vi "StepApproach.vi"() -> ()   [LabVIEW 2014]
uses:
  <vilib>/rvi/eio/common/nirviEmuTemplateMethod_errors.vi
  <vilib>/rvi/Emulation/niFpgaGetClockAttributes.vi
  <vilib>/rvi/Emulation/niFpgaSctlEmulationGetInTimedLoop.vi
  <vilib>/rvi/Emulation/niFpgaEmulationReportErrorSimple.vi
  <vilib>/rvi/Emulation/niFpgaCriticalErrorInLSC.vi
  <vilib>/rvi/Emulation/niFpgaProcessEmulError.vi
  <vilib>/rvi/interface/RandomDataEmulation/niFpgaRandomDataHandleErrors.vi
  <vilib>/eio/EIONode/EIONode.xnode
  <vilib>/rvi/DataTransferAndStorage/Container/XNode/niFpgaContainer.xnode
  <vilib>/rvi/interface/RandomDataEmulation/nirviRandomDataFpgaReadWriteTemplate.vi
panel:
  out "Numeric":i16
  out "PresentCount":i32
  in  "MeasureCount":i16
  in  "SeveralSampleMeasure?":bool
  in  "WithdrawStep":i16
  out "Result":bool
  out "PIZPosIndexDia":i16(graph)
  out "PreCurrIndexDia":i16(graph)
  out "PIZMaxPosIndex":i16
  out "PIZPosIndex":i16
  in  "stop":bool
  out "Approached?":bool
  in  "Offset":i16
  in  "AppRate us":u32
  out "RealPosIndex":i16
  out "preCurrIndex":i16
  in  "Percentage %":sgl format="%#_13g"
  in  "CurrSampleNum":u32
  in  "BaseTime us":u32
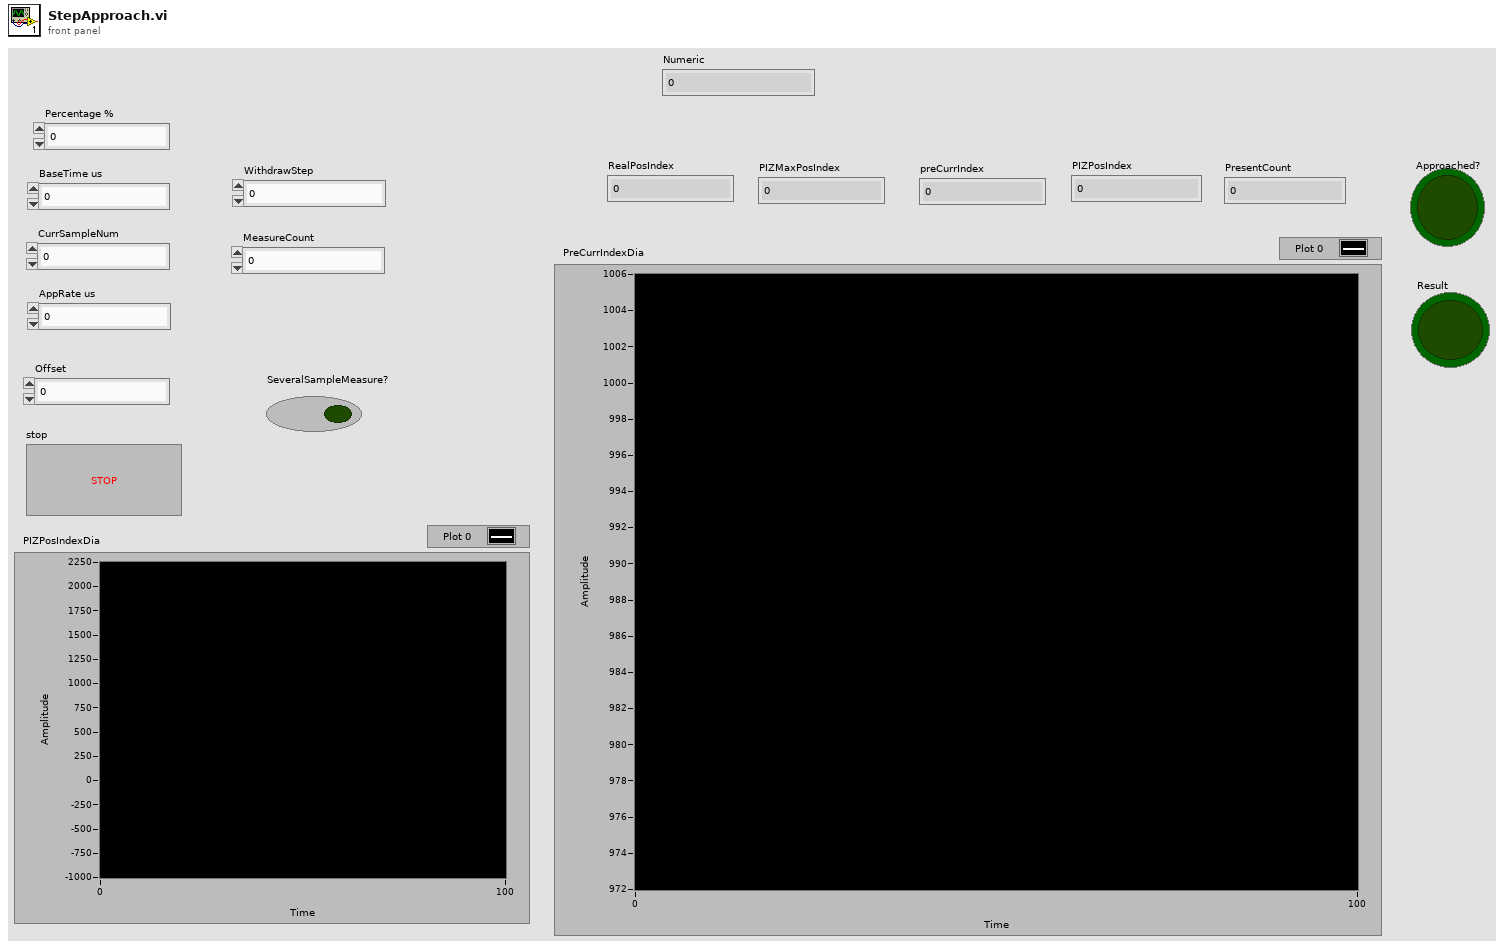
[diagram p1: front panel]
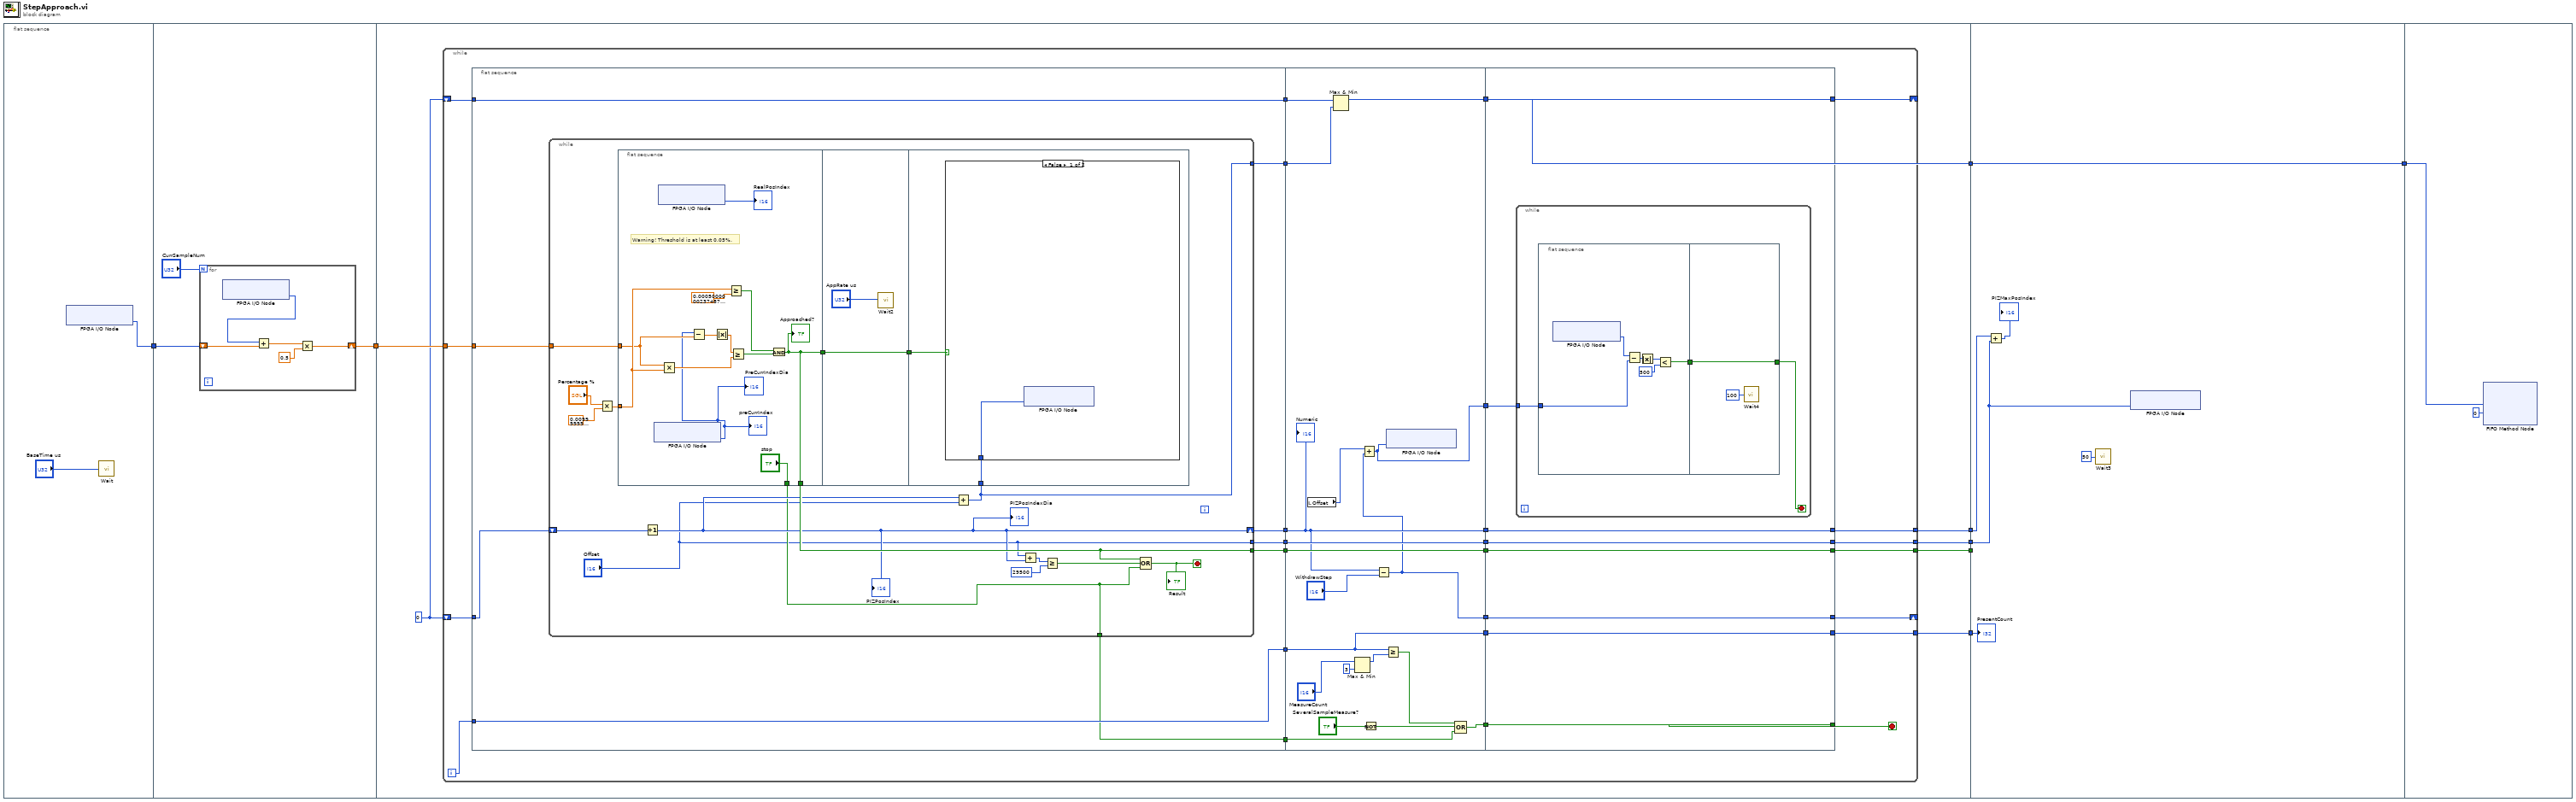
[diagram p0: block diagram]
diagram:
  n1 = flat-sequence {
    tunnel: [w9] -> w8
    tunnel: w8 -> [w12]
    tunnel: [w11] -> w7
    tunnel: w7 -> [w25]
    tunnel: [w24] -> w6
    tunnel: [w23] -> w5
    tunnel: [w22] -> w4
    tunnel: [w20] -> w3
    tunnel: [w21] -> w1
    tunnel: w6 -> [_]
    tunnel: w5 -> [w134]
    tunnel: w4 -> [w135]
    tunnel: w3 -> [w137]
    tunnel: [w137] -> w2
    tunnel: w1 -> [w132]
    tunnel: w2 -> [w139]
    frame #0 {
      n2 = xnode "FPGA I/O Node"() -> ("Connector0/AI1"=w9:i16)  [unwired: 1 in, 1 out]
      n3 = call "Wait"("Count(uSec)"="BaseTime us") -> ()  [unwired: 1 out]
    }
    frame #1 {
      n4 = for {
        N: "CurrSampleNum" -> [_]
        shift-right: [w14] -> w11
        shift-left: w12 -> [w17]
        n5 = xnode "FPGA I/O Node"() -> ("Connector0/AI1"=w18:i16)  [unwired: 1 in, 1 out]
        n6 = Add(x=w18, y=w17) -> (x+y=w16:sgl)
        n7 = Multiply(x=w16, y=sgl 0.5) -> (x*y=w14:sgl)
      }
    }
    frame #2 {
      w19 = i16 0
      n8 = while {
        tunnel: w25 -> [w51]
        tunnel: [w50] -> w24
        tunnel: [w49] -> w23
        tunnel: [w48] -> w22
        shift-right: [w43] -> _
        shift-left: w19 -> [w42]
        tunnel: [w38] -> w21
        shift-right: [w36] -> w20
        shift-left: w19 -> [w35]
        i -> [w41]
        stop <- w39 stop-if-true
        n9 = flat-sequence {
          tunnel: w51 -> [w60]
          tunnel: w42 -> [w52]
          tunnel: [w59] -> w47
          tunnel: [w58] -> w46
          tunnel: [w57] -> w45
          tunnel: [w56] -> w44
          tunnel: w41 -> [w55]
          tunnel: [w55] -> w40
          tunnel: w35 -> [w54]
          tunnel: [w54] -> w37
          tunnel: [w53] -> w27
          tunnel: w47 -> [w112]
          tunnel: w46 -> [w111]
          tunnel: w45 -> [w110]
          tunnel: w44 -> [w102]
          tunnel: w40 -> [w104]
          tunnel: w37 -> [w103]
          tunnel: [w112] -> w34
          tunnel: [w111] -> w33
          tunnel: [w110] -> w32
          tunnel: [w95] -> w31
          tunnel: [w98] -> w30
          tunnel: [w104] -> w29
          tunnel: [w101] -> w28
          tunnel: w27 -> [w97]
          tunnel: [w94] -> w26
          tunnel: [w115] -> w36
          tunnel: [w116] -> w38
          tunnel: [w117] -> w39
          tunnel: [w114] -> w43
          tunnel: [w118] -> w48
          tunnel: [w119] -> w49
          tunnel: [w120] -> w50
          tunnel: w34 -> [w120]
          tunnel: w33 -> [w119]
          tunnel: w32 -> [w118]
          tunnel: w31 -> [w114]
          tunnel: w30 -> [w117]
          tunnel: w29 -> [w116]
          tunnel: w28 -> [w115]
          tunnel: w26 -> [w113]
          frame #0 {
            n10 = while {
              tunnel: w60 -> [w76]
              shift-right: [w68] -> w57
              shift-left: w52 -> [w73]
              tunnel: [w72] -> w59
              tunnel: ["Offset"] -> w58
              tunnel: [w64] -> w56
              tunnel: [w62] -> w53
              stop <- w63 stop-if-true
              n11 = Multiply(x="Percentage %", y=sgl 0.01) -> (x*y=w65:sgl)
              n12 = flat-sequence {
                tunnel: w76 -> [w78]
                tunnel: [w83] -> w75
                tunnel: [w83] -> w72
                tunnel: ["stop"] -> w62
                tunnel: w65 -> [w81]
                tunnel: w75 -> [w90]
                tunnel: [w90] -> w74
                tunnel: w74 -> [w92]
                tunnel: w64 -> [w91]
                frame #0 {
                  # "Warning! Threshold is at least 0.05%."
                  n13 = xnode "FPGA I/O Node"() -> ("Connector0/AI1"=w77:i16)  [unwired: 1 in, 1 out]
                  "preCurrIndex" <- w77
                  "PreCurrIndexDia" <- w77
                  n14 = xnode "FPGA I/O Node"() -> ("Connector0/AI0"=→"RealPosIndex":i16)  [unwired: 1 in, 1 out]
                  n15 = Multiply(x=w78, y=w81) -> (x*y=w86:sgl)
                  n16 = Subtract(x=w77, y=w78) -> (x-y=w88:sgl)
                  n17 = Absolute Value(x=w88) -> (abs(x)=w87:sgl)
                  n18 = Greater Or Equal?(x=w81, y=sgl 0.0005) -> (x >= y?=w79:bool)
                  n19 = Greater Or Equal?(x=w87, y=w86) -> (x >= y?=w82:bool)
                  n20 = And(x=w79, y=w82) -> (x .and. y?=w83:bool)
                  "Approached?" <- w83
                }
                frame #1 {
                  n21 = call "Wait2"("Count(uSec)"="AppRate us") -> ()  [unwired: 1 out]
                }
                frame #2 {
                  n22 = case shown="False" w92 {
                    tunnel: w91 -> [w93 _]
                    frame False {
                      n23 = xnode "FPGA I/O Node"("Connector0/AO0"=w93) -> ()  [unwired: 1 in, 1 out]
                    }
                    frame True {
                    }
                  }
                }
              }
              n24 = Increment(x=w73) -> (x+1=w68:i16)
              "PIZPosIndex" <- w68
              "PIZPosIndexDia" <- w68
              n25 = Add(x=w68, y="Offset") -> (x+y=w64:i16)
              n26 = Add(x="Offset", y=w68) -> (x+y=w69:i16)
              n27 = Greater Or Equal?(x=w69, y=i16 29500) -> (x >= y?=w71:bool)
              n28 = Compound Arithmetic op=OR(w72, w71, w62) -> (w63:bool)
              "Result" <- w63
            }
          }
          frame #1 {
            n29 = local read "Offset"() -> (w96:i16)
            n30 = Max & Min(x=w103, y=w102) -> (max(x,y)=w101:i16)  [unwired: 1 out]
            n31 = Max & Min(x="MeasureCount", y=i16 3) -> (max(x,y)=w105:i16)  [unwired: 1 out]
            n32 = Not(x="SeveralSampleMeasure?") -> (.not. x?=w100:bool)
            n33 = Subtract(x=w110, y="WithdrawStep") -> (x-y=w95:i16)
            n34 = Add(x=w96, y=w95) -> (x+y=w94:i16)
            n35 = Greater Or Equal?(x=w104, y=w105) -> (x >= y?=w99:bool)
            n36 = xnode "FPGA I/O Node"("Connector0/AO0"=w94) -> ()  [unwired: 1 in, 1 out]
            n37 = Compound Arithmetic op=OR(w99, w100, w97) -> (w98:bool)
            "Numeric" <- w110
          }
          frame #2 {
            n38 = while {
              tunnel: w113 -> [w123]
              stop <- w122 stop-if-true
              n39 = flat-sequence {
                tunnel: w123 -> [w128]
                tunnel: [w126] -> w121
                tunnel: [w131] -> w122
                tunnel: w121 -> [w131]
                frame #0 {
                  n40 = xnode "FPGA I/O Node"() -> ("Connector0/AI0"=w129:i16)  [unwired: 1 in, 1 out]
                  n41 = Subtract(x=w129, y=w128) -> (x-y=w125:i16)
                  n42 = Absolute Value(x=w125) -> (abs(x)=w124:i16)
                  n43 = Less?(x=w124, y=i16 500) -> (x < y?=w126:bool)
                }
                frame #1 {
                  n44 = call "Wait4"("Count(uSec)"=u32 100) -> ()  [unwired: 1 out]
                }
              }
            }
          }
        }
      }
    }
    frame #3 {
      n45 = Add(x=w135, y=w134) -> (x+y=→"PIZMaxPosIndex":i16)
      n46 = call "Wait3"("Count(uSec)"=u32 50) -> ()  [unwired: 1 out]
      n47 = xnode "FPGA I/O Node"("Connector0/AO0"=w134) -> ()  [unwired: 1 in, 1 out]
      "PresentCount" <- w132
    }
    frame #4 {
      n48 = xnode ("FIFO Method Node")("Element"=w139, "Timeout"=0) -> ()  [unwired: 1 in, 2 out]
    }
  }
